vi "Initialize Configuration Display.vi"(8 "error in (no error)":errorcluster, 10 "Configuration Pane References":T1, 11 "Configuration in":refnum<class "Configuration.lvclass">) -> (0 "error out":errorcluster, 1 "Stop Event Loop":refnum<user-event>, 2 "Change Display":refnum<user-event>, 3 "Configuration out":refnum<class "Configuration.lvclass">)   [LabVIEW 2016, in "Configuration.lvlib" / "Configuration.lvclass"]
uses:
  <userlib>/Configuration Dialog Actor/Configuration.lvclass
  C:/Program Files (x86)/National Instruments/LabVIEW 2016/vi.lib/ActorFramework/Actor/Actor.lvclass
  <userlib>/Configuration Dialog Actor/Methods/Config Actor Core UI Ref.ctl
  <userlib>/Configuration Dialog Actor/Configuration.lvclass/Configuration.ctl
  <vilib>/ActorFramework/Actor/Actor.lvclass/Actor.ctl
  <vilib>/ActorFramework/Message Enqueuer/Message Enqueuer.lvclass/Message Enqueuer.ctl
  <userlib>/Configuration Dialog Actor/Configuration Messages/Display New Configuration SubPanel Msg/Display New Configuration SubPanel Msg.lvclass/Display New Configuration SubPanel Msg.ctl
  <vilib>/ActorFramework/Message Enqueuer/Init from Existing Queue.vi
  <vilib>/ActorFramework/Message Enqueuer/Enqueue.vi
  <userlib>/Configuration Dialog Actor/Configuration Messages/Display New Configuration SubPanel Msg/Display New Configuration SubPanel Msg.lvclass
  C:/Program Files (x86)/National Instruments/LabVIEW 2016/vi.lib/ActorFramework/Message/Message.lvclass
  <vilib>/ActorFramework/Message Priority Queue/Priority Enqueue.vi
  <vilib>/ActorFramework/Message Enqueuer/Message Enqueuer.lvclass
  <vilib>/ActorFramework/Actor/Actor.lvclass
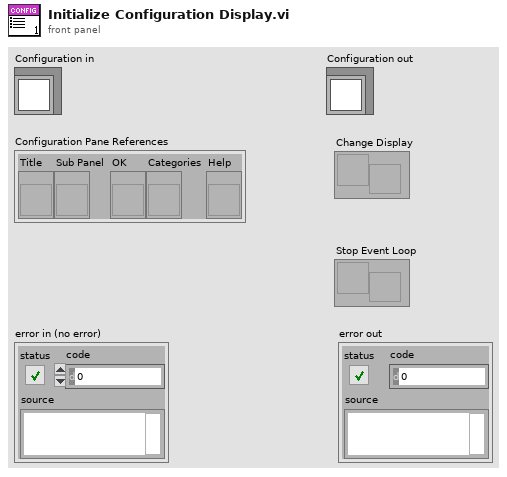
[diagram p1: front panel]
types:
  T1 = typedef "Configuration.lvlib/Configuration.lvclass/Config Actor Core UI Ref.ctl" = cluster{"Title":refnum<vi>, "Sub Panel":refnum<vi>, "OK":refnum<vi>, "Categories":refnum<vi>, "Help":refnum<vi>}
  T2 = enum16{"Alphabetical Ascending", "Alphabetical Descending", "Chronological", "Reverse Chronological"}
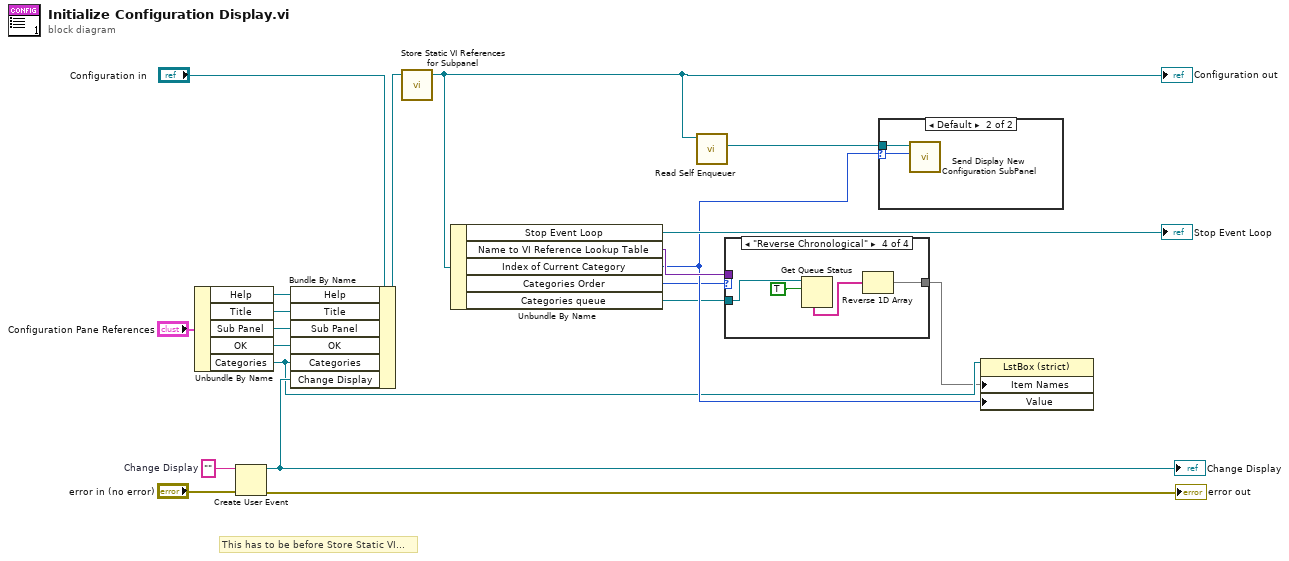
[diagram p0: block diagram]
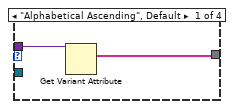
[diagram p2: hidden frame]
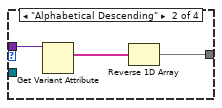
[diagram p3: hidden frame]
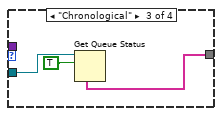
[diagram p4: hidden frame]
diagram:
  w19 = ""  # Change Display
  # "This has to be before Store Static VI..."
  n1 = Unbundle By Name("Configuration Pane References") -> ("Help"=w11:refnum<vi>, "Title"=w15:refnum<vi>, "Sub Panel"=w14:refnum<vi>, "OK"=w13:refnum<vi>, "Categories"=w7:refnum<vi>)
  n2 = Create User Event(user event datatype=w19, error in="error in (no error)") -> (user event=w20:refnum<user-event>, error out=→"error out":errorcluster)
  "Change Display" <- w20
  n3 = Bundle By Name(cluster="Configuration in", "Help"=w11, "Title"=w15, "Sub Panel"=w14, "OK"=w13, "Categories"=w7, "Change Display"=w20) -> (w5:refnum<class "Configuration.lvclass">)
  n4 = call-dynamic "Store Static VI References for Subpanel.vi"("Configuration in"=w5) -> ("Configuration out"=w4:refnum<class "Configuration.lvclass">)  [unwired: 9 in, 1 out]
  "Configuration out" <- w4
  n5 = Unbundle By Name(w4) -> ("Stop Event Loop"=→"Stop Event Loop":refnum<user-event>, "Name to VI Reference Lookup Table"=w18:variant, "Index of Current Category"=w9:i32, "Categories Order"=w3:T2, "Categories queue"=w1:refnum<queue>)
  n6 = call <vilib>:"Read Self Enqueuer.vi"("Actor"=w4) -> ("Self Enqueuer"=w10:refnum<class "Message Enqueuer.lvclass">)  [unwired: 10 in]
  n7 = case shown="\"Reverse Chronological\"" w3 {
    tunnel: w18 -> [w22 w25 _ _]
    tunnel: [w21 w23 w26 w29] -> w2
    tunnel: w1 -> [_ _ w28 w31]
    frame "Alphabetical Ascending", Default {
      n8 = Get Variant Attribute(Variant=w22) -> (names=w21:string[])  [unwired: 3 in, 3 out]
    }
    frame "Alphabetical Descending" {
      n9 = Get Variant Attribute(Variant=w25) -> (names=w24:string[])  [unwired: 3 in, 3 out]
      n10 = Reverse 1D Array(array=w24) -> (reversed array=w23:string[])
    }
    frame "Chronological" {
      n11 = Get Queue Status(queue=w28, return elements? (F)=TRUE) -> (elements=w26:string[])  [unwired: 1 in, 7 out]
    }
    frame "Reverse Chronological" {
      n12 = Get Queue Status(queue=w31, return elements? (F)=TRUE) -> (elements=w30:string[])  [unwired: 1 in, 7 out]
      n13 = Reverse 1D Array(array=w30) -> (reversed array=w29:string[])
    }
  }
  n14 = case shown="Default" w9 {
    selector: w9 -> [_ w33]
    tunnel: w10 -> [_ w34]
    frame -1 {
    }
    frame Default {
      n15 = call <userlib>:"Send Display New Configuration SubPanel.vi"("ListBox Selection"=w33, "Message Enqueuer"=w34) -> ()  [unwired: 8 in, 2 out]
    }
  }
  n16 = property class="LstBox (strict)"(reference=w7, "Item Names"=w2, "Value"=w9) -> ()  [unwired: 1 in, 2 out]
